vi "3458A CALSTR Panel.vi"(8 "error in (no error)":errorcluster, 11 "VISA":refnum<visa-resource-name> caption="VISA resource name") -> (0 "error out":errorcluster)   [LabVIEW 2020, in "3458A Virtual Digitizer.lvlib"]
doc: "Simple GUI for reading and writing CALSTR to 3458A."
uses:
  3458A Virtual Digitizer.lvlib
  3458A Digitizing Low Levels/3458A Digitizing Low Levels.lvlib
  3458A Basic Driver/3458A Basic Driver.lvlib
panel:
  in  "CALCODE (default: 3458)":string="3458"
  in  "btn write":bool
  out "serial":string caption="Parsed serial number"
  in  "CALSTR data":string
  in  "btn read":bool
  in  "btn exit":bool
  in  "btn id":bool
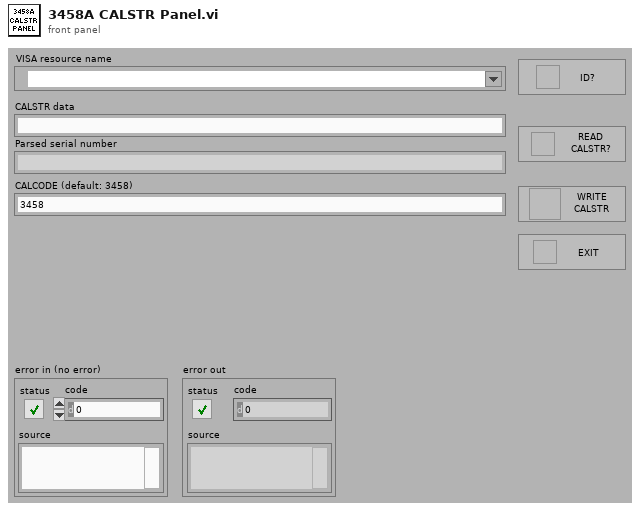
[diagram p1: front panel]
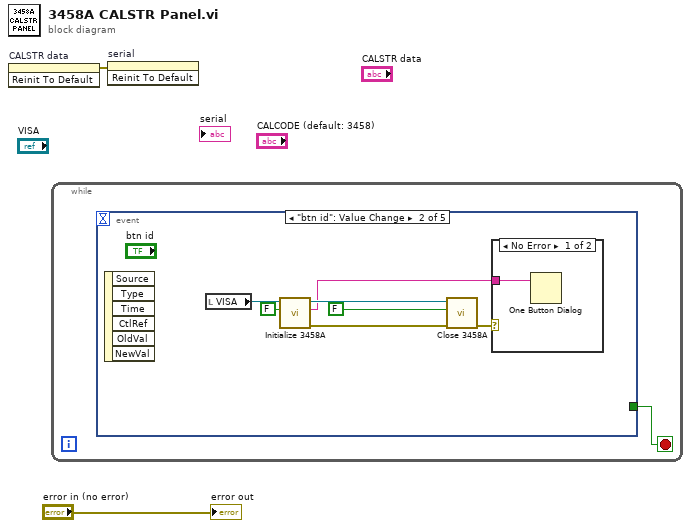
[diagram p0: block diagram]
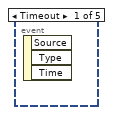
[diagram p2: hidden frame]
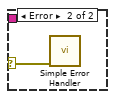
[diagram p3: hidden frame]
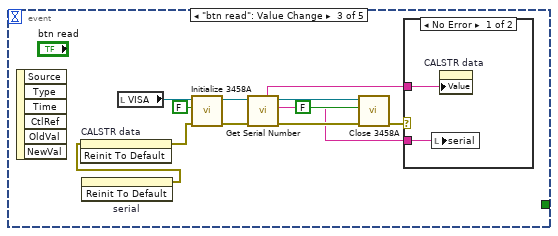
[diagram p4: hidden frame]
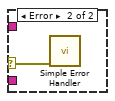
[diagram p5: hidden frame]
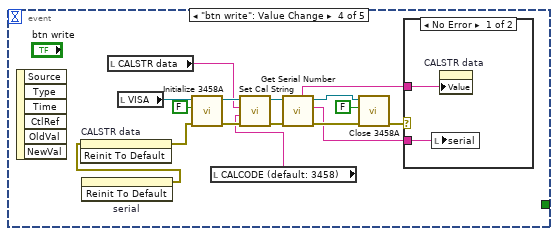
[diagram p6: hidden frame]
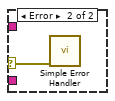
[diagram p7: hidden frame]
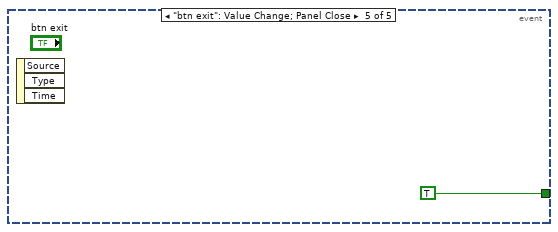
[diagram p8: hidden frame]
diagram:
  n1 = invoke on="CALSTR data" class="Str" method="Reinit To Default"() -> (error out=w1:errorcluster)  [unwired: 3 in, 2 out]
  n2 = while {
    stop <- w3 stop-if-true
    n3 = event shown="[1] \"btn id\": Value Change" {
      selector: _ -> [_ _ _ _ _]
      dyn-events: _ -> [_ _ _ _ _]
      timeout: _ -> [_ _ _ _ _]
      tunnel: [_ _ _ _ TRUE] -> w3
      event Timeout {
        n4 = event-data() -> ()  [unwired: 1 in, 3 out]
      }
      event "btn id": Value Change {
        n5 = event-data() -> ()  [unwired: 1 in, 6 out]
        n6 = local read "VISA"() -> (w10:refnum<visa-resource-name>)
        n7 = call "Initialize 3458A.vi"("Reset (True)"=FALSE, "VISA DMM"=w10) -> ("error out"=w9:errorcluster, "idn string"=w4:string, "VISA resource name out"=w8:refnum<visa-resource-name>)  [unwired: 6 in, 1 out]
        n8 = call "Close 3458A.vi"("error in (no error)"=w9, "Reset to preset mode (True)"=FALSE, "VISA resource name"=w8) -> ("error out"=w5:errorcluster)  [unwired: 8 in]
        n9 = case shown="No Error" w5 {
          selector: w5 -> [_ w12]
          tunnel: w4 -> [w11 _]
          frame No Error {
            n10 = One Button Dialog(message=w11) -> ()  [unwired: 1 in, 1 out]
          }
          frame Error {
            n11 = call <vilib>:"Simple Error Handler.vi"("error in (no error)"=w12) -> ()  [unwired: 4 in, 5 out]
          }
        }
      }
      event "btn read": Value Change {
        n12 = event-data() -> ()  [unwired: 1 in, 6 out]
        n13 = invoke on="serial" class="Str" method="Reinit To Default"() -> (error out=w14:errorcluster)  [unwired: 3 in, 2 out]
        n14 = invoke on="CALSTR data" class="Str" method="Reinit To Default"(error in=w14) -> (error out=w20:errorcluster)  [unwired: 2 in, 2 out]
        n15 = local read "VISA"() -> (w24:refnum<visa-resource-name>)
        n16 = call "Initialize 3458A.vi"("error in (no error)"=w20, "Reset (True)"=FALSE, "VISA DMM"=w24) -> ("error out"=w19:errorcluster, "VISA resource name out"=w18:refnum<visa-resource-name>)  [unwired: 5 in, 2 out]
        n17 = call "Get Serial Number.vi"("error in"=w19, "VISA resource in"=w18) -> ("error out"=w17:errorcluster, "serial number"=w13:string, "VISA resource out"=w16:refnum<visa-resource-name>, "CALSTR"=w15:string)  [unwired: 5 in, 1 out]
        n18 = call "Close 3458A.vi"("error in (no error)"=w17, "Reset to preset mode (True)"=FALSE, "VISA resource name"=w16) -> ("error out"=w21:errorcluster)  [unwired: 8 in]
        n19 = case shown="No Error" w21 {
          selector: w21 -> [_ w27]
          tunnel: w15 -> [w26 _]
          tunnel: w13 -> [w25 _]
          frame No Error {
            n20 = local write "serial"(w25) -> ()
            n21 = property on="CALSTR data" class="Str"("Value"=w26) -> ()  [unwired: 2 in, 2 out]
          }
          frame Error {
            n22 = call <vilib>:"Simple Error Handler.vi"("error in (no error)"=w27) -> ()  [unwired: 4 in, 5 out]
          }
        }
      }
      event "btn write": Value Change {
        n23 = event-data() -> ()  [unwired: 1 in, 6 out]
        n24 = invoke on="serial" class="Str" method="Reinit To Default"() -> (error out=w36:errorcluster)  [unwired: 3 in, 2 out]
        n25 = invoke on="CALSTR data" class="Str" method="Reinit To Default"(error in=w36) -> (error out=w39:errorcluster)  [unwired: 2 in, 2 out]
        n26 = local read "CALSTR data"() -> (w35:string)
        n27 = local read "VISA"() -> (w43:refnum<visa-resource-name>)
        n28 = call "Initialize 3458A.vi"("error in (no error)"=w39, "Reset (True)"=FALSE, "VISA DMM"=w43) -> ("error out"=w38:errorcluster, "VISA resource name out"=w37:refnum<visa-resource-name>)  [unwired: 5 in, 2 out]
        n29 = local read "CALCODE (default: 3458)"() -> (w28:string)
        n30 = call "Set Cal String.vi"("error in(no error)"=w38, "calcode"=w28, "calibration string"=w35, "VISA Resource Name"=w37) -> ("error out"=w34:errorcluster, "VISA resource name out"=w33:refnum<visa-resource-name>)  [unwired: 6 in]
        n31 = call "Get Serial Number.vi"("error in"=w34, "VISA resource in"=w33) -> ("error out"=w32:errorcluster, "serial number"=w29:string, "VISA resource out"=w31:refnum<visa-resource-name>, "CALSTR"=w30:string)  [unwired: 5 in, 1 out]
        n32 = call "Close 3458A.vi"("error in (no error)"=w32, "Reset to preset mode (True)"=FALSE, "VISA resource name"=w31) -> ("error out"=w40:errorcluster)  [unwired: 8 in]
        n33 = case shown="No Error" w40 {
          selector: w40 -> [_ w46]
          tunnel: w30 -> [w45 _]
          tunnel: w29 -> [w44 _]
          frame No Error {
            n34 = local write "serial"(w44) -> ()
            n35 = property on="CALSTR data" class="Str"("Value"=w45) -> ()  [unwired: 2 in, 2 out]
          }
          frame Error {
            n36 = call <vilib>:"Simple Error Handler.vi"("error in (no error)"=w46) -> ()  [unwired: 4 in, 5 out]
          }
        }
      }
      event "btn exit": Value Change; Panel Close {
        n37 = event-data() -> ()  [unwired: 1 in, 3 out]
      }
    }
  }
  n38 = invoke on="serial" class="Str" method="Reinit To Default"(error in=w1) -> ()  [unwired: 2 in, 3 out]
  "error out" <- "error in (no error)"
